vi "Get Charact Type.vi"(11 "error in (no error)":errorcluster) -> (4 "Charact type":string, 15 "error out":errorcluster)   [LabVIEW 2023, in "RFFixtureCharact.Public.lvlib"]
uses:
  RFFixtureCharact.Public.lvlib
  Common/Data Cache/Settings Dictionary/Setting Keys.vi
  Common/RFCalAndFixtureCharact.Common.lvlib
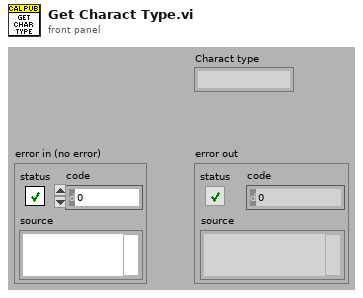
[diagram p1: front panel]
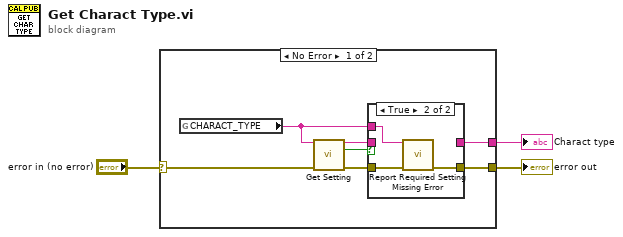
[diagram p0: block diagram]
diagram:
  n1 = case shown="No Error" "error in (no error)" {
    selector: "error in (no error)" -> [w10 w16]
    tunnel: [w7 w16] -> w2
    tunnel: [w4 _] -> w1
    frame No Error {
      n2 = global read "Setting Keys.vi" "CHARACT_TYPE"() -> (w9:string)
      n3 = call "Get Setting.vi"("Setting name"=w9, "error in (no error)"=w10) -> ("Setting value out"=w5:string, "Setting empty or not found?"=w6:bool, "error out"=w8:errorcluster)  [unwired: 11 in]
      n4 = case shown="True" w6 {
        tunnel: [w12 w14] -> w7
        tunnel: w8 -> [w12 w15]
        tunnel: w9 -> [_ w13]
        tunnel: w5 -> [w11 _]
        tunnel: [w11 _] -> w4
        frame False {
        }
        frame True {
          n5 = call "Report Required Setting Missing Error.vi"("Setting name"=w13, "Error in (no error)"=w15) -> ("error out"=w14:errorcluster)  [unwired: 13 in]
        }
      }
    }
    frame Error {
    }
  }
  "error out" <- w2
  "Charact type" <- w1
